vi "sub_Synchronize_Packet.vi"(6 "Realign Waveform (T)":bool=TRUE, 9 "Sync Sequence Waveform":cdb[](array[numeric]), 10 "Expected Sync Index":i32, 11 "Input Complex Waveform":T1={"t0"=0.0, "dt"=1.0, "Y"=[]} {"Y" format="%.3f"; "dt" format="%^.2e"; "t0" format="%.4f"}) -> (0 "Xcorr Waveform":cdb[](array[numeric]), 1 "Frame Offset (samples)":i32, 2 "Max Xcorr Index":i32, 3 "Output Complex Waveform":T1={"t0"=0.0, "dt"=1.0, "Y"=[]} {"Y" format="%.3f"; "dt" format="%^.2e"; "t0" format="%.4f"})   [LabVIEW 2014]
uses:
  <vilib>/addons/Modulation/Analog/controls/Complex Data Waveform.ctl
  <vilib>/Analysis/2dsp.llb/1D Cross Correlation (CDB).vi
  <vilib>/Analysis/NI_AALPro.lvlib
  <vilib>/addons/Modulation/niAMT.lvlib
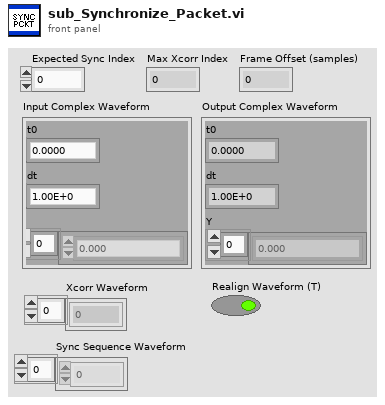
[diagram p1: front panel]
types:
  T1 = typedef "niAMT.lvlib/Complex Data Waveform.ctl" = cluster{"t0":dbl, "dt":dbl, "Y":cdb[]}
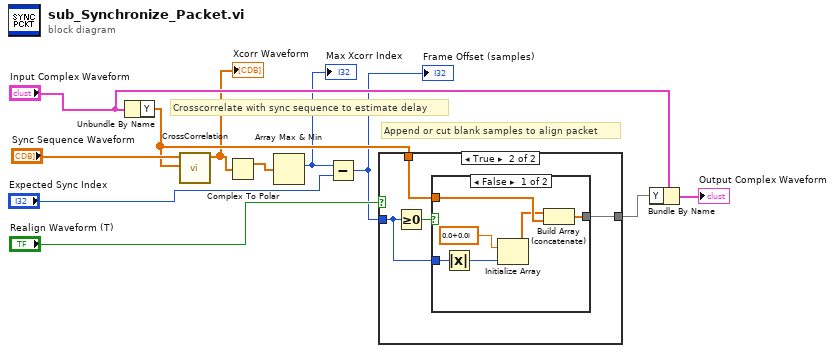
[diagram p0: block diagram]
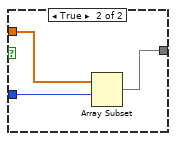
[diagram p3: hidden frame]
diagram:
  # "Append or cut blank samples to align packet"
  # "Crosscorrelate with sync sequence to estimate delay"
  n1 = Unbundle By Name("Input Complex Waveform") -> ("Y"=w6:cdb[])
  n2 = call-poly <vilib>:"CrossCorrelation.vi"("Y"=w6, "X"="Sync Sequence Waveform") -> ("Rxy"=w2:cdb[])  [unwired: 8 in, 1 out]
  "Xcorr Waveform" <- w2
  n3 = Complex To Polar(r * e^(i*theta)=w2) -> (r=w1:dbl[])  [unwired: 1 out]
  n4 = Array Max & Min(array=w1) -> (max index (indices)=w4:i32)  [unwired: 3 out]
  "Max Xcorr Index" <- w4
  n5 = Subtract(x=w4, y="Expected Sync Index") -> (x-y=w5:i32)
  "Frame Offset (samples)" <- w5
  n6 = case shown="True" "Realign Waveform (T)" {
    tunnel: [w12 w16] -> w3
    tunnel: w5 -> [_ w14]
    tunnel: w6 -> [w12 w15]
    frame False {
    }
    frame True {
      n7 = Greater Or Equal To 0?(x=w14) -> (x >= 0?=w13:bool)
      n8 = case shown="False" w13 {
        tunnel: [w17 w25] -> w16
        tunnel: w15 -> [w19 w24]
        tunnel: w14 -> [w22 w23]
        frame False {
          n9 = Absolute Value(x=w22) -> (abs(x)=w21:i32)
          n10 = Initialize Array(cdb 0.0+0.0i ("element"), w21) -> (w18:cdb[])
          n11 = Build Array (concatenate)(w18, w19) -> (w17:cdb[])
        }
        frame True {
          n12 = Array Subset(array=w24, index=w23) -> (w25:cdb[])  [unwired: 1 in]
        }
      }
    }
  }
  n13 = Bundle By Name(cluster="Input Complex Waveform", "Y"=w3) -> (→"Output Complex Waveform":T1)
